vi "main - 20131122-1045.vi"() -> ()   [LabVIEW 2013]
uses:
  states.ctl
  <vilib>/Instr/_visa.llb/VISA Set IO Buffer Mask.ctl
  <vilib>/Instr/_visa.llb/VISA Configure Serial Port (Instr).vi
panel:
  out "StopRobot":bool
  in  "DelayTime":u32=100
  in  "baud rate (9600)":u32=9600 caption="波特率"
  in  "VISA resource name":refnum<visa-resource-name> caption="VISA资源名称"
  out "RoCmdString":string
  in  "StopFour":bool
  in  "ClockWise":bool
  in  "AntiClockWise":bool
  in  "Up":bool
  in  "Down":bool
  in  "StopButton":bool
  in  "States":T1
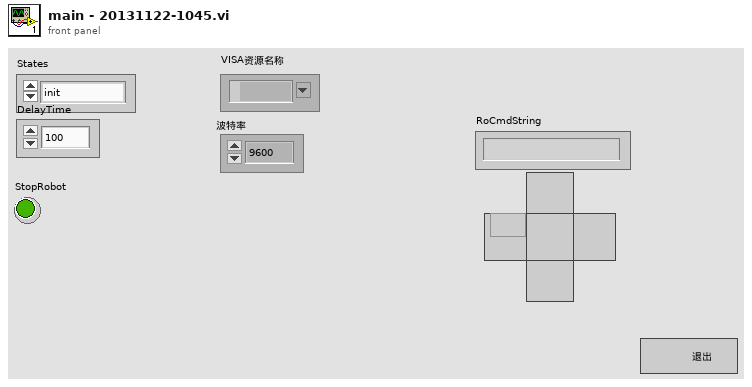
[diagram p1: front panel]
types:
  T1 = typedef "states.ctl" = enum16{"init", "wait", "stop", "ro-up", "ro-down", "ro-clockwise", "ro-anticlockwise", "ro-stopstaut"}
  T2 = typedef "VISA Set IO Buffer Mask.ctl" = u16
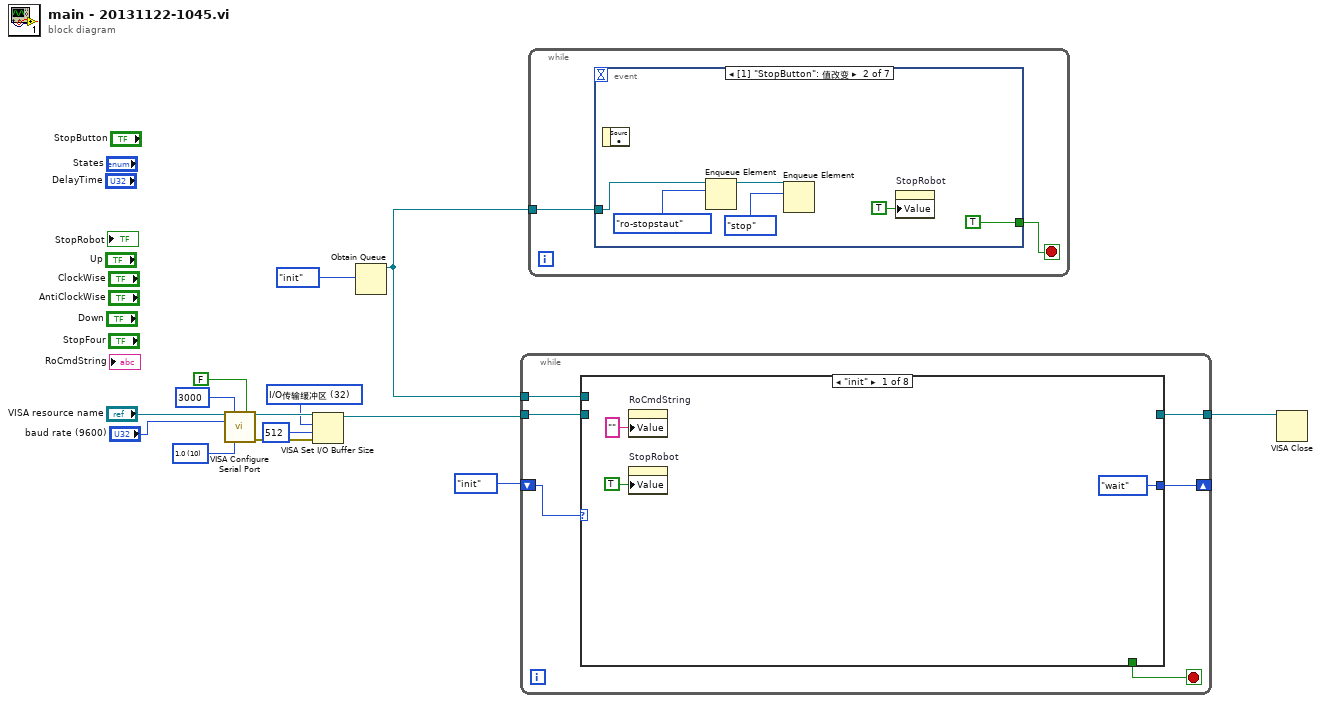
[diagram p0: block diagram]
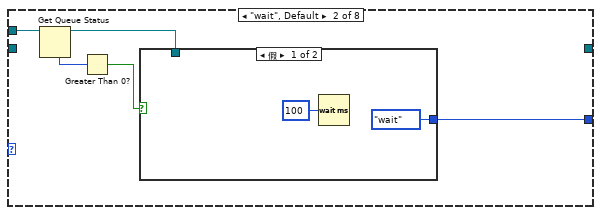
[diagram p2: hidden frame]
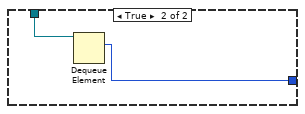
[diagram p3: hidden frame]
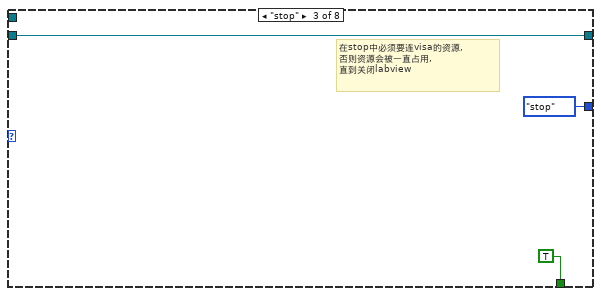
[diagram p4: hidden frame]
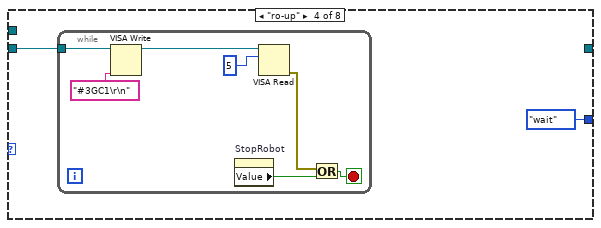
[diagram p5: hidden frame]
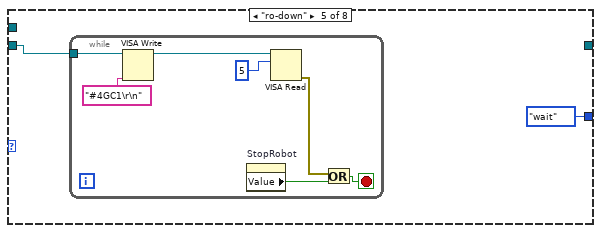
[diagram p6: hidden frame]
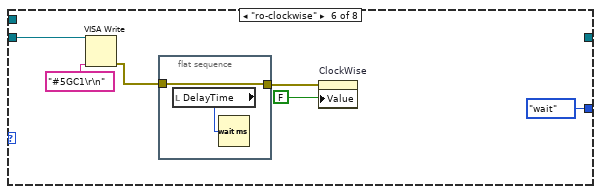
[diagram p7: hidden frame]
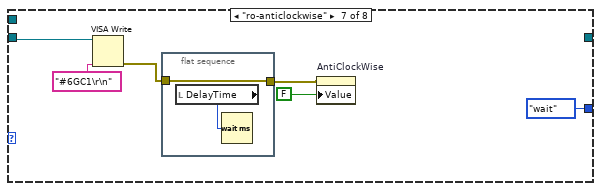
[diagram p8: hidden frame]
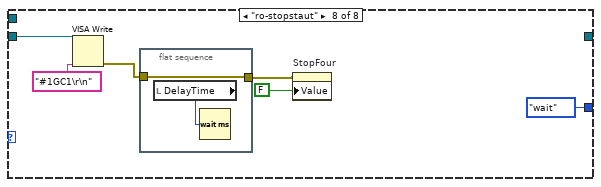
[diagram p9: hidden frame]
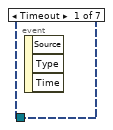
[diagram p10: hidden frame]
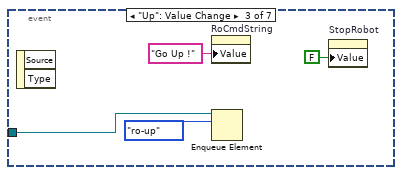
[diagram p11: hidden frame]
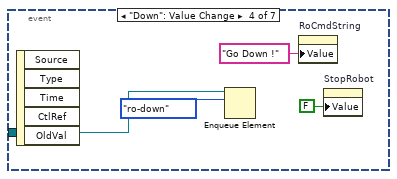
[diagram p12: hidden frame]
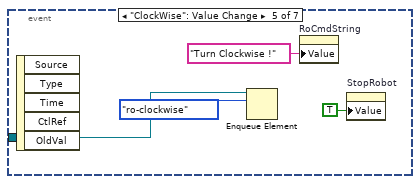
[diagram p13: hidden frame]
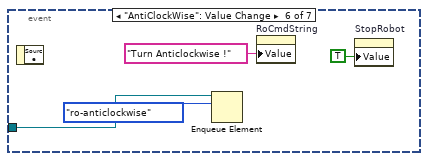
[diagram p14: hidden frame]
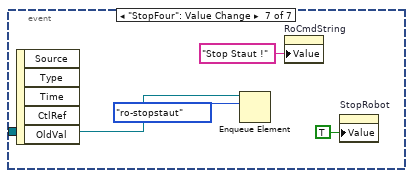
[diagram p15: hidden frame]
diagram:
  w4 = T2 32 items=["I/O接收缓冲区"=16, "I/O传输缓冲区"=32, "I/O接收和传输缓冲区"=48] ("Mask")
  w8 = u16 10 items=["1.0"=10, "1.5"=15, "2.0"=20] ("stop bits (10: 1 bit)")
  n1 = call-poly "VISA Configure Serial Port"("VISA resource name"="VISA resource name", "timeout (10sec)"=u32 3000, "Enable Termination\nChar (T)"=FALSE ("Enable Termination\nChar (T)"), "baud rate (9600)"="baud rate (9600)", "stop bits (10: 1 bit)"=w8) -> ("VISA resource name out"=w6:refnum<visa-resource-name>, "error out"=w2:errorcluster)  [unwired: 9 in]
  n2 = VISA Set I/O Buffer Size(VISA resource name=w6, mask (16)=w4, size (4096)=u32 512 ("大小(4096)"), error in (no error)=w2) -> (VISA resource name out=w5:refnum<visa-resource-name>)  [unwired: 1 out]
  n3 = Obtain Queue(element data type=states."init" ("States")) -> (queue out=w14:refnum<queue>)  [unwired: 4 in, 2 out]
  n4 = while {
    tunnel: w14 -> [w18]
    shift-right: [w17] -> _
    shift-left: states."init" ("States") -> [w20]
    tunnel: w5 -> [w16]
    tunnel: [w15] -> w7
    stop <- w19 stop-if-true
    n5 = case shown="\"init\"" w20 {
      tunnel: [_ _ TRUE _ _ _ _ _] -> w19
      tunnel: w18 -> [_ w28 _ _ _ _ _ _]
      tunnel: [states."wait" ("States") w24 states."stop" ("States") states."wait" ("States") states."wait" ("States") states."wait" ("States") states."wait" ("States") states."wait" ("States")] -> w17
      tunnel: w16 -> [_ _ w33 w36 w45 w58 w66 w74]
      tunnel: [_ _ w33 _ _ _ _ _] -> w15
      frame "init" {
        n6 = property on="RoCmdString" class="Str"("Value"="" ("RoCmdString")) -> ()  [unwired: 2 in, 2 out]
        n7 = property on="StopRobot" class="Bool (严格)"("Value"=TRUE ("StopRobot")) -> ()  [unwired: 2 in, 2 out]
      }
      frame "wait", Default {
        n8 = Get Queue Status(queue=w28) -> (queue out=w25:refnum<queue>, # elements in queue=w27:i32)  [unwired: 2 in, 6 out]
        n9 = Greater Than 0?(x=w27) -> (x > 0?=w26:bool)
        n10 = case shown="假" w26 {
          tunnel: w25 -> [_ w32]
          tunnel: [states."wait" ("States") w31] -> w24
          frame False {
            n11 = Wait (ms)(milliseconds to wait=u32 100 ("等待时间（毫秒）")) -> ()  [unwired: 1 out]
          }
          frame True {
            n12 = Dequeue Element(queue=w32) -> (element=w31:T1)  [unwired: 2 in, 3 out]
          }
        }
      }
      frame "stop" {
        # "在stop中必须要连visa的资源,\n否则资源会被一直占用,\n直到关闭labview"
      }
      frame "ro-up" {
        n13 = while {
          tunnel: w36 -> [w43]
          stop <- w38 stop-if-true
          n14 = VISA Write(VISA resource name=w43, write buffer="#3GC1\r\n" ("写入缓冲区")) -> (VISA resource name out=w41:refnum<visa-resource-name>)  [unwired: 1 in, 2 out]
          n15 = property on="StopRobot" class="Bool (严格)"() -> ("Value"=w39:bool)  [unwired: 2 in, 2 out]
          n16 = VISA Read(VISA resource name=w41, byte count=u32 5 ("字节总数")) -> (error out=w40:errorcluster)  [unwired: 1 in, 3 out]
          n17 = Or(x=w40, y=w39) -> (x .or. y?=w38:bool)
        }
      }
      frame "ro-down" {
        n18 = while {
          tunnel: w45 -> [w52]
          stop <- w47 stop-if-true
          n19 = VISA Write(VISA resource name=w52, write buffer="#4GC1\r\n" ("写入缓冲区")) -> (VISA resource name out=w50:refnum<visa-resource-name>)  [unwired: 1 in, 2 out]
          n20 = property on="StopRobot" class="Bool (严格)"() -> ("Value"=w48:bool)  [unwired: 2 in, 2 out]
          n21 = VISA Read(VISA resource name=w50, byte count=u32 5 ("字节总数")) -> (error out=w49:errorcluster)  [unwired: 1 in, 3 out]
          n22 = Or(x=w49, y=w48) -> (x .or. y?=w47:bool)
        }
      }
      frame "ro-clockwise" {
        n23 = VISA Write(VISA resource name=w58, write buffer="#5GC1\r\n" ("写入缓冲区")) -> (error out=w55:errorcluster)  [unwired: 1 in, 2 out]
        n24 = flat-sequence {
          tunnel: [w61] -> w56
          tunnel: w55 -> [w61]
          frame #0 {
            n25 = local read "DelayTime"() -> (w60:u32)
            n26 = Wait (ms)(milliseconds to wait=w60) -> ()  [unwired: 1 out]
          }
        }
        n27 = property on="ClockWise" class="Bool (严格)"(error in=w56, "Value"=FALSE ("Up")) -> ()  [unwired: 1 in, 2 out]
      }
      frame "ro-anticlockwise" {
        n28 = VISA Write(VISA resource name=w66, write buffer="#6GC1\r\n" ("写入缓冲区")) -> (error out=w62:errorcluster)  [unwired: 1 in, 2 out]
        n29 = flat-sequence {
          tunnel: [w69] -> w63
          tunnel: w62 -> [w69]
          frame #0 {
            n30 = local read "DelayTime"() -> (w68:u32)
            n31 = Wait (ms)(milliseconds to wait=w68) -> ()  [unwired: 1 out]
          }
        }
        n32 = property on="AntiClockWise" class="Bool (严格)"(error in=w63, "Value"=FALSE ("Up")) -> ()  [unwired: 1 in, 2 out]
      }
      frame "ro-stopstaut" {
        n33 = VISA Write(VISA resource name=w74, write buffer="#1GC1\r\n" ("写入缓冲区")) -> (error out=w70:errorcluster)  [unwired: 1 in, 2 out]
        n34 = flat-sequence {
          tunnel: [w77] -> w72
          tunnel: w70 -> [w77]
          frame #0 {
            n35 = local read "DelayTime"() -> (w76:u32)
            n36 = Wait (ms)(milliseconds to wait=w76) -> ()  [unwired: 1 out]
          }
        }
        n37 = property on="StopFour" class="Bool (严格)"(error in=w72, "Value"=FALSE ("Up")) -> ()  [unwired: 1 in, 2 out]
      }
    }
  }
  n38 = while {
    tunnel: w14 -> [w79]
    stop <- w78 stop-if-true
    n39 = event shown="[1] \"StopButton\": 值改变" {
      selector: _ -> [_ _ _ _ _ _ _]
      dyn-events: _ -> [_ _ _ _ _ _ _]
      timeout: _ -> [_ _ _ _ _ _ _]
      tunnel: w79 -> [_ w81 w88 w92 w96 w100 w103]
      tunnel: [_ TRUE _ _ _ _ _] -> w78
      event Timeout {
        n40 = event-data() -> ()  [unwired: 1 in, 3 out]
      }
      event "StopButton": Value Change {
        n41 = event-data() -> ()  [unwired: 1 in, 1 out]
        n42 = Enqueue Element(queue=w81, element=states."ro-stopstaut" ("States")) -> (queue out=w80:refnum<queue>)  [unwired: 2 in, 2 out]
        n43 = Enqueue Element(queue=w80, element=states."stop" ("States")) -> ()  [unwired: 2 in, 3 out]
        n44 = property on="StopRobot" class="Bool (严格)"("Value"=TRUE ("StopRobot")) -> ()  [unwired: 2 in, 2 out]
      }
      event "Up": Value Change {
        n45 = event-data() -> ()  [unwired: 1 in, 2 out]
        n46 = property on="RoCmdString" class="Str"("Value"="Go Up !" ("RoCmdString")) -> ()  [unwired: 2 in, 2 out]
        n47 = Enqueue Element(queue=w88, element=states."ro-up" ("States")) -> ()  [unwired: 2 in, 3 out]
        n48 = property on="StopRobot" class="Bool (严格)"("Value"=FALSE ("StopRobot")) -> ()  [unwired: 2 in, 2 out]
      }
      event "Down": Value Change {
        n49 = event-data() -> ()  [unwired: 1 in, 5 out]
        n50 = Enqueue Element(queue=w92, element=states."ro-down" ("States")) -> ()  [unwired: 2 in, 3 out]
        n51 = property on="RoCmdString" class="Str"("Value"="Go Down !" ("RoCmdString")) -> ()  [unwired: 2 in, 2 out]
        n52 = property on="StopRobot" class="Bool (严格)"("Value"=FALSE ("StopRobot")) -> ()  [unwired: 2 in, 2 out]
      }
      event "ClockWise": Value Change {
        n53 = event-data() -> ()  [unwired: 1 in, 5 out]
        n54 = Enqueue Element(queue=w96, element=states."ro-clockwise" ("States")) -> ()  [unwired: 2 in, 3 out]
        n55 = property on="RoCmdString" class="Str"("Value"="Turn Clockwise !" ("RoCmdString")) -> ()  [unwired: 2 in, 2 out]
        n56 = property on="StopRobot" class="Bool (严格)"("Value"=TRUE ("StopRobot")) -> ()  [unwired: 2 in, 2 out]
      }
      event "AntiClockWise": Value Change {
        n57 = event-data() -> ()  [unwired: 1 in, 1 out]
        n58 = Enqueue Element(queue=w100, element=states."ro-anticlockwise" ("States")) -> ()  [unwired: 2 in, 3 out]
        n59 = property on="RoCmdString" class="Str"("Value"="Turn Anticlockwise !" ("RoCmdString")) -> ()  [unwired: 2 in, 2 out]
        n60 = property on="StopRobot" class="Bool (严格)"("Value"=TRUE ("StopRobot")) -> ()  [unwired: 2 in, 2 out]
      }
      event "StopFour": Value Change {
        n61 = event-data() -> ()  [unwired: 1 in, 5 out]
        n62 = Enqueue Element(queue=w103, element=states."ro-stopstaut" ("States")) -> ()  [unwired: 2 in, 3 out]
        n63 = property on="RoCmdString" class="Str"("Value"="Stop Staut !" ("RoCmdString")) -> ()  [unwired: 2 in, 2 out]
        n64 = property on="StopRobot" class="Bool (严格)"("Value"=TRUE ("StopRobot")) -> ()  [unwired: 2 in, 2 out]
      }
    }
  }
  n65 = VISA Close(VISA resource name=w7) -> ()  [unwired: 1 in, 1 out]
